vi "GPIB_Write.vi"(0 "address string":string, 1 "data In":string, 2 "mode (0)":i16, 3 "error in":errorcluster, 4 "timeout ms (488.2 global)":i32=2000) -> (5 "status":bool[](array[boolean]), 6 "error out":errorcluster)   [LabVIEW 2010]
uses:
  Controls/GPIB_Mode.ctl
  Globals/Preference_global.vi
  Globals/Dynamic_call_global.ph.vi
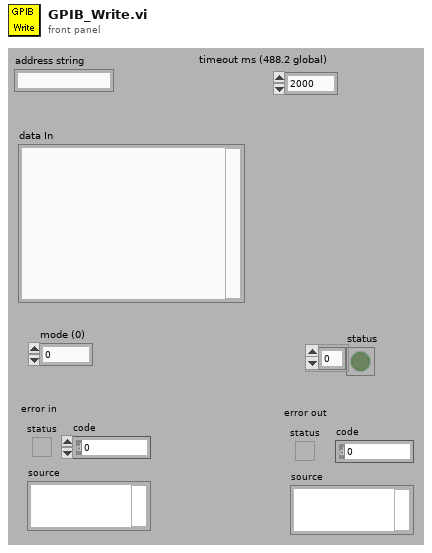
[diagram p1: front panel]
types:
  T1 = typedef "GPIB_Mode.ctl" = enum16{"Read", "Write", "Trigger", "Poll"}
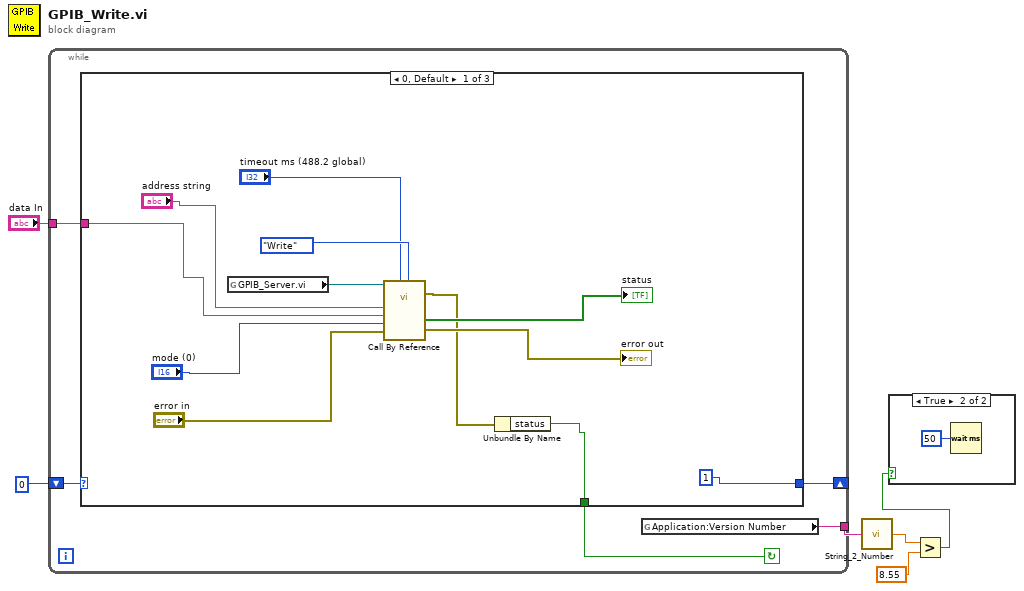
[diagram p0: block diagram]
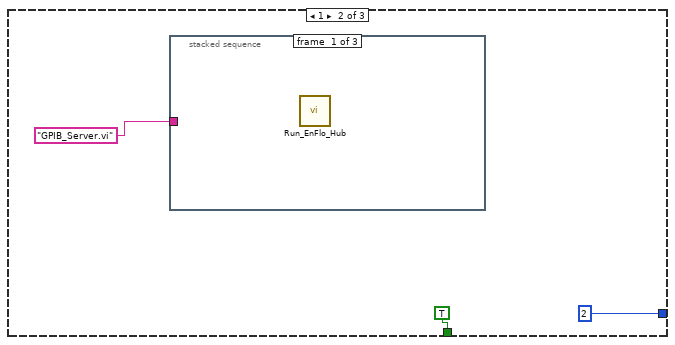
[diagram p3: hidden frame]
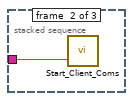
[diagram p4: hidden frame]
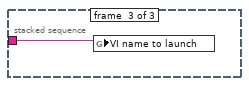
[diagram p5: hidden frame]
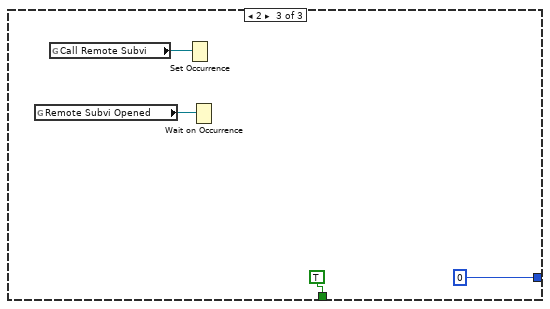
[diagram p6: hidden frame]
diagram:
  n1 = while {
    shift-right: [w10] -> _
    shift-left: 0 -> [w11]
    tunnel: "data In" -> [w8]
    tunnel: [w7] -> w4
    stop <- w9 continue-if-true
    n2 = case shown="0, Default" w11 {
      tunnel: [1 2 0] -> w10
      tunnel: [w22 TRUE ("status") TRUE ("status")] -> w9
      tunnel: w8 -> [w21 _ _]
      frame 0, Default {
        n3 = global read "Dynamic_call_global.ph.vi" "GPIB_Server.vi"() -> (w20:refnum<vi>)
        n4 = call-by-ref "?"(reference=w20, "Case"=GPIB_Mode."Write", "error in"="error in", "mode (0)"="mode (0)", "timeout ms (488.2 global)"="timeout ms (488.2 global)", "data In"=w21, "address string"="address string") -> (error out=w12:errorcluster, 0:"error out"=→"error out":errorcluster, "status"=→"status":bool[])  [unwired: 3 in, 2 out]
        n5 = Unbundle By Name(w12) -> ("status"=w22:bool)
      }
      frame 1 {
        n6 = stacked-sequence {
          tunnel: "GPIB_Server.vi" ("VI name to launch") -> [_ w27 w28]
          frame #0 {
            n7 = call "Run_EnFlo_Hub.vi"() -> ()  [unwired: 8 out]
          }
          frame #1 {
            n8 = call "Start_Client_Coms.vi"("VI name to run on server"=w27) -> ()  [unwired: 1 in, 4 out]
          }
          frame #2 {
            n9 = global write "Dynamic_call_global.ph.vi" "VI name to launch"(w28) -> ()
          }
        }
      }
      frame 2 {
        n10 = global read "Dynamic_call_global.ph.vi" "Remote Subvi Opened"() -> (w31:refnum<k4>)
        n11 = global read "Dynamic_call_global.ph.vi" "Call Remote Subvi"() -> (w32:refnum<k4>)
        n12 = Set Occurrence(w32) -> ()
        n13 = Wait on Occurrence(2:w31) -> ()  [unwired: 3 out]
      }
    }
    n14 = global read "Preference_global.vi" "Application:Version Number"() -> (w7:string)
  }
  n15 = call "String_2_Number.vi"("Value"=w4) -> ("Numeric"=w3:dbl)
  n16 = Greater?(x=w3, y=8.55) -> (0:w1:bool)
  n17 = case shown="True" w1 {
    frame False {
    }
    frame True {
      n18 = Wait (ms)(milliseconds to wait=u32 50) -> ()  [unwired: 1 out]
    }
  }
